vi "LV to ITX  Retrieve.vi"(0 "File or Folder Path":path=path "C:/", 1 "Data Type":T1=enum."DAT", 2 "DAT header length":i32=11, 5 "offset":i32, 7 "length":i32=1, 9 "index":T2={"A"=1, "B"=0, "C"=2, "D"=0, "E"=3, "N1"=0, "N2"=0, "N3"=0, "N4"=0}, 11 "error in (no error)":errorcluster) -> (4 "A vs B":cluster{dbl[], dbl[]}[](graph), 6 "C vs D":cluster{dbl[], dbl[]}[](graph), 8 "E":dbl[][](graph), 10 "N":cluster{"N1":dbl, "N2":dbl, "N3":dbl, "N4":dbl}={"N1"=0.0624995231628418, "N2"=0.0624995231628418, "N3"=0.0624995231628418, "N4"=0.0624995231628418} {"N4" format="%#_6p"; "N3" format="%#_6p"; "N2" format="%#_6p"; "N1" format="%#_6p"}, 14 "Notes":string)   [LabVIEW 2019, in "LV-Data.ITX.lvclass"]
uses:
  LV-Data.ITX.lvclass
  <vilib>/Utility/miscctls.llb/LVOffsetAndMultiplierTypeDef.ctl
  Typedefs/Retrieve Data Type.ctl
  LV-Data/LV-Data.lvclass
  <userlib>/LevyLab/Graph Utilities/graph_utilities.lvclass
panel:
  in  "D  is time?":bool
  in  "B is time?":bool
  out "time":string[][](table)
  in  "Use Folder Index File?":bool
  in  "Generate Folder Index File?":bool
  in  "Ez name":string="Ez name"
  in  "Ey name":string="Ey name"
  in  "Ex name":string="Ex name"
  in  "C y name":string="C y name"
  in  "D x name":string="D x name"
  in  "A y name":string="A y name"
  in  "B x name":string="B x name"
  out "Index, Wavenames":string[][](table)
  in  "recolor traces?":bool
  in  "Ex":T3={"Offset"=0.0, "Multiplier"=1.0}
  in  "Ey":T3={"Offset"=0.0, "Multiplier"=1.0}
  out "Path":path
  out "counter":i32
  out "pattern":string="*.dat"
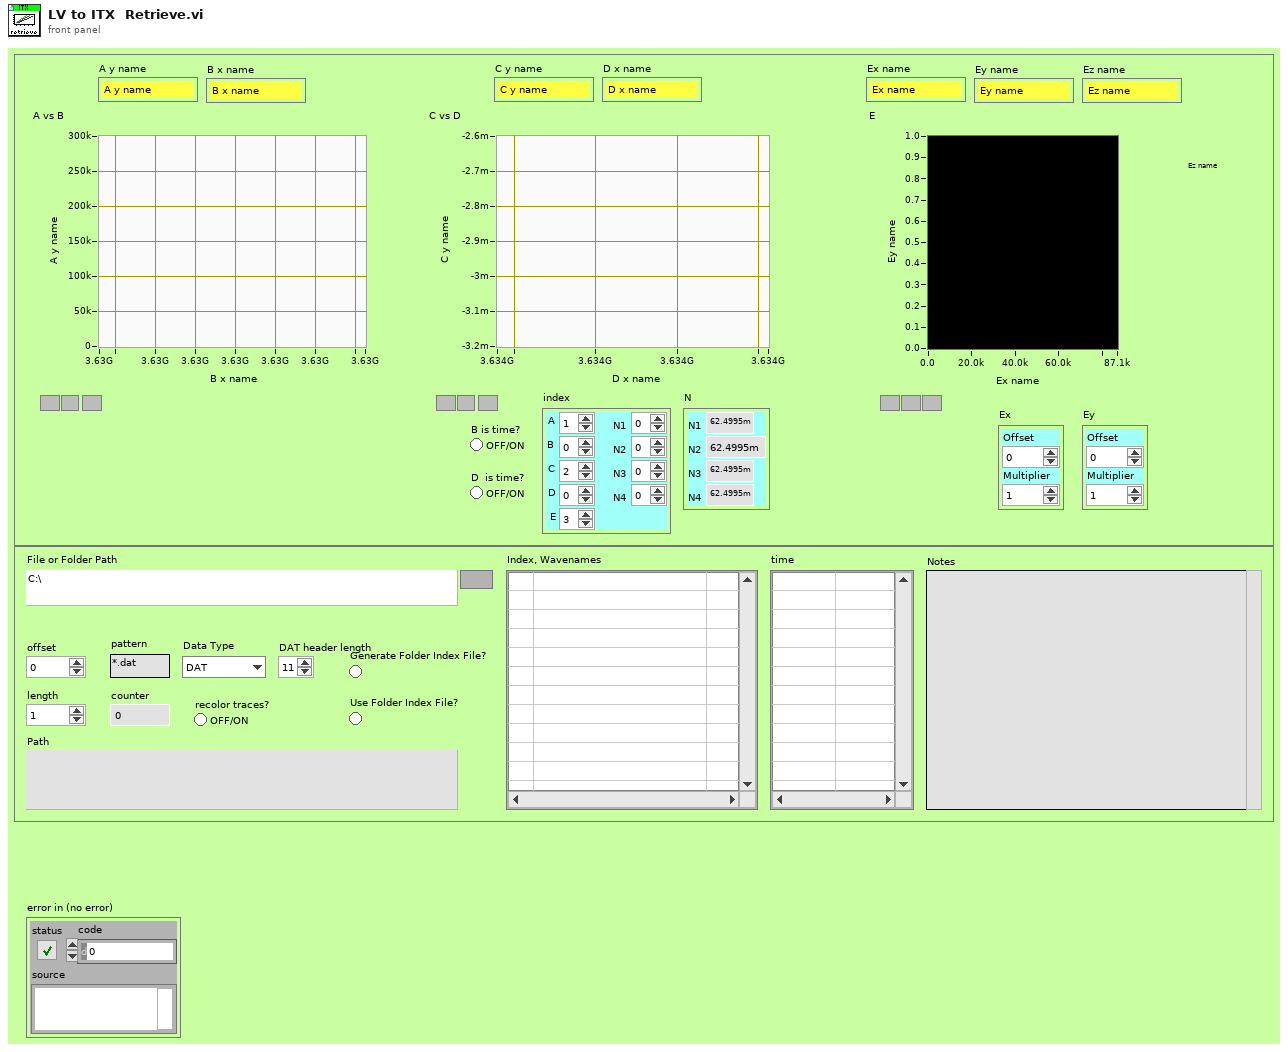
[diagram p1: front panel]
types:
  T1 = typedef "LV-Data.ITX.lvclass/Retrieve Data Type.ctl" = enum16{"ITX", "ITX w/ 2D", "DAT", "TDMS"}
  T2 = cluster{"A":i32, "B":i32, "C":i32, "D":i32, "E":i32, "N1":i32, "N2":i32, "N3":i32, "N4":i32}
  T3 = typedef "LVOffsetAndMultiplierTypeDef.ctl" = cluster{"Offset":dbl, "Multiplier":dbl}
  T4 = typedef "LV-Data.lvclass/Dictionary--cluster.ctl" = cluster{"key":string, "value":variant}
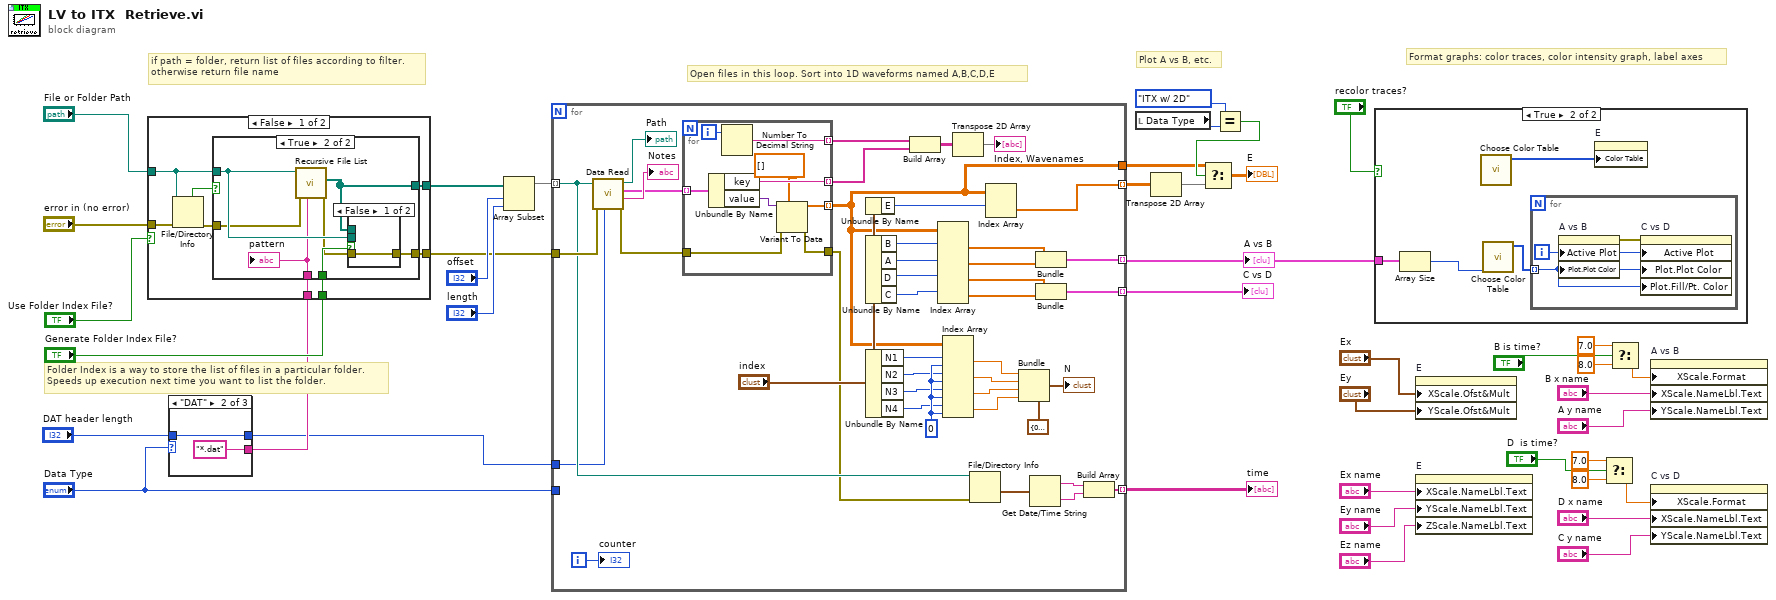
[diagram p0: block diagram]
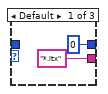
[diagram p2: hidden frame]
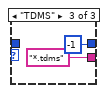
[diagram p3: hidden frame]
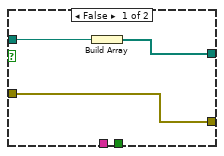
[diagram p5: hidden frame]
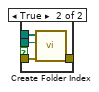
[diagram p6: hidden frame]
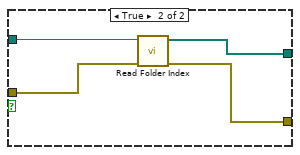
[diagram p7: hidden frame]
diagram:
  # "Plot A vs B, etc."
  # "Format graphs: color traces, color intensity graph, label axes"
  # "Open files in this loop. Sort into 1D waveforms named A,B,C,D,E"
  # "Folder Index is a way to store the list of files in a particular folder.\nSpeeds up execution next time you want to list the folder."
  # "if path = folder, return list of files according to filter.\notherwise return file name"
  n1 = case shown="\"DAT\"" "Data Type" {
    tunnel: ["*.itx" ("pattern") "*.dat" ("pattern") "*.tdms" ("pattern")] -> w7
    tunnel: "DAT header length" -> [_ w44 _]
    tunnel: [0 ("DAT header length") w44 -1 ("DAT header length")] -> w1
    frame Default {
    }
    frame "DAT" {
    }
    frame "TDMS" {
    }
  }
  n2 = case shown="False" "Use Folder Index File?" {
    tunnel: [w53 w73] -> w39
    tunnel: "File or Folder Path" -> [w55 w74]
    tunnel: "Generate Folder Index File?" -> [w52 _]
    tunnel: w7 -> [w51 _]
    tunnel: "error in (no error)" -> [w50 w72]
    tunnel: [w48 w71] -> w4
    frame False {
      n3 = File/Directory Info(path=w55, error in=w50) -> (directory=w54:bool, error out=w49:errorcluster)  [unwired: 5 out]
      n4 = case shown="True" w54 {
        tunnel: [w58 w64] -> w53
        tunnel: w55 -> [w57 w65]
        tunnel: w52 -> [_ w62]
        tunnel: w51 -> [_ w63]
        tunnel: w49 -> [w56 w60]
        tunnel: [w56 w61] -> w48
        frame False {
          n5 = Build Array(w57) -> (w58:path[])
        }
        frame True {
          n6 = call <vilib>:"Recursive File List.vi"("pattern"=w63, "error in (no error)"=w60, "Folder Path"=w65) -> ("error out"=w59:errorcluster, "All Files in Dir"=w64:path[])  [unwired: 4 in, 3 out]
          n7 = case shown="False" w62 {
            tunnel: w64 -> [_ w70]
            tunnel: w65 -> [_ w69]
            tunnel: w59 -> [w66 w68]
            tunnel: [w66 w67] -> w61
            frame False {
            }
            frame True {
              n8 = call "Create Folder Index.vi"("error in (no error)"=w68, "File or Folder Path"=w69, "All Files in Dir"=w70) -> ("error out"=w67:errorcluster)  [unwired: 8 in]
            }
          }
          "pattern" <- w63
        }
      }
    }
    frame True {
      n9 = call "Read Folder Index.vi"("error in (no error)"=w72, "File or Folder Path"=w74) -> ("error out"=w71:errorcluster, "Files"=w73:path[])  [unwired: 8 in]
    }
  }
  n10 = Array Subset(array=w39, index="offset", length="length") -> (w19:path[])
  n11 = for {
    tunnel: w19 -> [w86] mode=indexing
    tunnel: [w115] -> w31 mode=indexing
    tunnel: [w114] -> w30 mode=indexing
    tunnel: [w78] -> w34 mode=indexing
    tunnel: [w79] -> w3
    tunnel: [w91] -> w22 mode=indexing
    tunnel: "Data Type" -> [_]
    tunnel: w1 -> [w75]
    tunnel: w4 -> [w87]
    i -> [w116]
    w108 = 0 ("disabled index (col)")
    n12 = call "Data Read.vi"("Append Index"=w75, "error in (no error)"=w87, "path"=w86) -> ("error out"=w81:errorcluster, "Notes"=→"Notes":string, "Data (Dictionary)"=w83:T4[], "path out"=→"Path":path)  [unwired: 5 in]
    n13 = for {
      tunnel: [w124] -> w112 mode=indexing
      tunnel: w83 -> [w123] mode=indexing
      tunnel: [w122] -> w82 mode=indexing
      tunnel: [w120] -> w79 mode=indexing
      tunnel: w81 -> [w118]
      tunnel: [w117] -> w80
      i -> [w125]
      n14 = Unbundle By Name(w123) -> ("key"=w122:string, "value"=w119:variant)
      n15 = Number To Decimal String(number=w125) -> (decimal integer string=w124:string)  [unwired: 1 in]
      n16 = Variant To Data(error in=w118, type=dbl[] [], Variant=w119) -> (data=w120:dbl[], error out=w117:errorcluster)
    }
    n17 = Unbundle By Name("index") -> ("E"=w102:i32)
    n18 = Unbundle By Name("index") -> ("B"=w101:i32, "A"=w100:i32, "D"=w99:i32, "C"=w98:i32)
    n19 = Unbundle By Name("index") -> ("N1"=w103:i32, "N2"=w77:i32, "N3"=w76:i32, "N4"=w104:i32)
    n20 = Build Array(w112, w82) -> (w109:string[][])
    n21 = Index Array(array=w79, index (row) #1=w101, index (row) #2=w100, index (row) #3=w99, index (row) #4=w98) -> (element #1=w96:dbl[], element #2=w95:dbl[], element #3=w110:dbl[], element #4=w113:dbl[])  [unwired: 4 in]
    n22 = Index Array(array=w79, index (row) #1=w103, index (col) #1=w108, index (row) #2=w77, index (col) #2=w108, index (row) #3=w76, index (col) #3=w108, index (row) #4=w104, index (col) #4=w108) -> (element #1=w92:dbl, element #2=w93:dbl, element #3=w94:dbl, element #4=w107:dbl)
    n23 = Transpose 2D Array(2D array=w109) -> (transposed array=→"Index, Wavenames":string[][])
    n24 = File/Directory Info(path=w86, error in=w80) -> (last mod=w90:timestamp)  [unwired: 6 out]
    n25 = Index Array(array=w79, index (row)=w102) -> (element=w78:dbl[])  [unwired: 1 in]
    n26 = Bundle(cluster=cluster{"N1":dbl, "N2":dbl, "N3":dbl, "N4":dbl} {"N1"=0.0, "N2"=0.0, "N3"=0.0, "N4"=0.0}, "N1"=w92, "N2"=w93, "N3"=w94, "N4"=w107) -> (→"N":cluster{"N1":dbl, "N2":dbl, "N3":dbl, "N4":dbl})
    n27 = Get Date/Time String(seconds (now)=w90) -> (date string=w88:string, time string=w89:string)  [unwired: 2 in]
    n28 = Bundle(w96, w95) -> (w115:cluster{dbl[], dbl[]})  [unwired: 1 in]
    n29 = Bundle(w110, w113) -> (w114:cluster{dbl[], dbl[]})  [unwired: 1 in]
    n30 = Build Array(w88, w89) -> (w91:string[])
    "counter" <- w116
  }
  "A vs B" <- w31
  "C vs D" <- w30
  "time" <- w22
  n31 = local read "Data Type"() -> (w10:T1)
  n32 = Transpose 2D Array(2D array=w34) -> (transposed array=w35:dbl[][])
  n33 = Equal?(x=enum16{"ITX", "ITX w/ 2D", "DAT"}."ITX w/ 2D" ("Enum"), y=w10) -> (x = y?=w8:bool)
  n34 = Select(t=w3, s=w8, f=w35) -> (s? t:f=→"E":dbl[][])
  n35 = case shown="True" "recolor traces?" {
    tunnel: w31 -> [_ w127]
    frame False {
    }
    frame True {
      n36 = Array Size(array=w127) -> (size(s)=w126:i32)
      n37 = call <userlib>:"Choose Color Table.vi"() -> ("Color Table"=w129:u32[])  [unwired: 8 in, 3 out]
      n38 = call <userlib>:"Choose Color Table.vi"("Size (256)"=w126) -> ("Color Table"=w128:u32[])  [unwired: 7 in, 3 out]
      n39 = for {
        tunnel: w128 -> [w130] mode=indexing
        i -> [w131]
        n40 = property on="A vs B" class="XYGraph (strict)"("Active Plot"=w131, "Plot.Plot Color"=w130) -> (error out=w132:errorcluster)  [unwired: 2 in, 1 out]
        n41 = property on="C vs D" class="XYGraph (strict)"(error in=w132, "Active Plot"=w131, "Plot.Plot Color"=w130, "Plot.Fill/Pt. Color"=w130) -> ()  [unwired: 1 in, 2 out]
      }
      n42 = property on="E" class="IntGraph (strict)"("Color Table"=w129) -> ()  [unwired: 2 in, 2 out]
    }
  }
  n43 = property on="E" class="IntGraph (strict)"("XScale.Ofst&Mult"="Ex", "YScale.Ofst&Mult"="Ey") -> ()  [unwired: 2 in, 2 out]
  n44 = property on="E" class="IntGraph (strict)"("XScale.NameLbl.Text"="Ex name", "YScale.NameLbl.Text"="Ey name", "ZScale.NameLbl.Text"="Ez name") -> ()  [unwired: 2 in, 2 out]
  n45 = Select(t=7.0, s="D  is time?", f=8.0) -> (s? t:f=w15:dbl)
  n46 = Select(t=7.0, s="B is time?", f=8.0) -> (s? t:f=w16:dbl)
  n47 = property on="A vs B" class="XYGraph (strict)"("XScale.Format"=w16, "XScale.NameLbl.Text"="B x name", "YScale.NameLbl.Text"="A y name") -> ()  [unwired: 2 in, 2 out]
  n48 = property on="C vs D" class="XYGraph (strict)"("XScale.Format"=w15, "XScale.NameLbl.Text"="D x name", "YScale.NameLbl.Text"="C y name") -> ()  [unwired: 2 in, 2 out]
